vi "string_to_dbl_SubVI.vi"(0 "input string":string, 3 "error in":errorcluster, 13 "max t in":i8) -> (2 "max t out":i8, 4 "T":dbl, 8 "T bool":bool, 14 "error out":errorcluster)   [LabVIEW 2013]
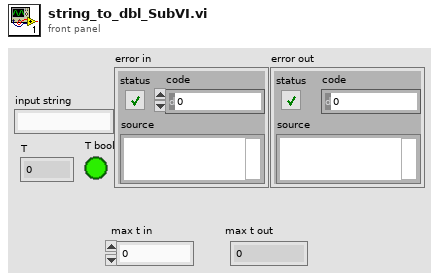
[diagram p1: front panel]
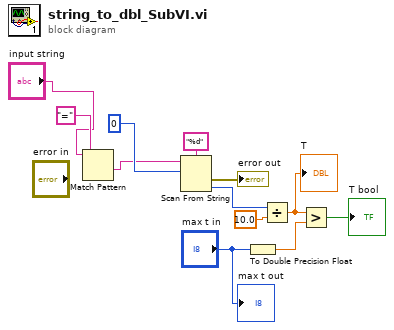
[diagram p0: block diagram]
diagram:
  n1 = Match Pattern(string="input string", regular expression="=") -> (after substring=w3:string)  [unwired: 1 in, 3 out]
  n2 = Scan From String(format string="%d", input string=w3, initial scan location=u32 0) -> (error out=→"error out":errorcluster, output 1=w10:i32)  [unwired: 2 in, 2 out]
  n3 = To Double Precision Float(number="max t in") -> (double precision float=w5:dbl)
  n4 = Divide(x=w10, y=10.0) -> (x/y=w6:dbl)
  "T" <- w6
  n5 = Greater?(x=w6, y=w5) -> (0:→"T bool":bool)
  "max t out" <- "max t in"
